vi "PV ActiveLine - Node address for 485.vi"(7 "W/R":bool, 8 "Fehler (Eingang)":errorcluster, 9 "Node address":u16=1 min=1 max=24 step=1, 11 "Referenz in":refnum<visa-resource-name>) -> (0 "Cluster (Ausgang)":errorcluster, 1 "Node address out":i8=1, 2 "Read Status":u16(ring) items=["Read Failed", "Read Ok"], 3 "Referenz out":refnum<visa-resource-name>)   [LabVIEW 2013, in "PV ActiveLine.lvlib"]
doc: "NAD - RS485 Node Address\n\nTransmit: NAD [,a]\nReceive: a\n\nRS485 node address,\na = 1 … 24"
uses:
  <instrlib>/PV ActiveLine/PV ActiveLine.lvlib
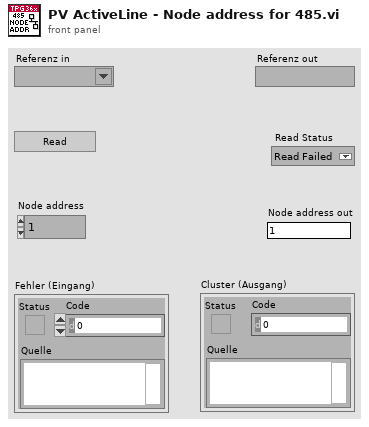
[diagram p1: front panel]
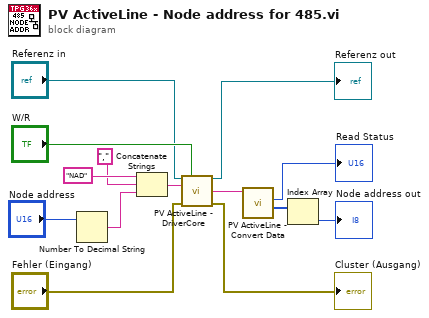
[diagram p0: block diagram]
diagram:
  n1 = Number To Decimal String(number="Node address") -> (decimal integer string=w12:string)  [unwired: 1 in]
  n2 = Concatenate Strings("NAD" ("Command"), "," ("Command"), w12) -> (w10:string)
  n3 = call <instrlib>:"PV ActiveLine - DriverCore.vi"("Referenz in"="Referenz in", "Write/Read"="W/R", "Command"=w10, "Fehler (Eingang)"="Fehler (Eingang)") -> ("Referenz out"=→"Referenz out":refnum<visa-resource-name>, "String Out"=w5:string, "Cluster (Ausgang)"=→"Cluster (Ausgang)":errorcluster)  [unwired: 9 in]
  n4 = call <instrlib>:"PV ActiveLine - Convert Data.vi"("String in"=w5) -> ("Integer Out"=w3:i32[], "Read Status"=→"Read Status":u16)  [unwired: 7 in, 2 out]
  n5 = Index Array(array=w3) -> (element=→"Node address out":i32)  [unwired: 1 in]
